vi "PNS Ausgabefelder einfaerben.vi"(6 "Aktionen":T1, 9 "maxLoop":i32=10, 11 "Angehängtes Array":refnum<vi>[](array[refnum])) -> ()   [LabVIEW 2020, in "PNS.lvlib" / "PNS Anlagenuebersicht.lvlib"]
uses:
  PNS Anlagenuebersicht.lvlib
  PNS Ausgabefelder einfaerben Aktionen.ctl
  Aktionen FGV Grenzwerte.ctl
  Allgemein/allgemeine Sub-VIs.lvlib
  PNS.lvlib
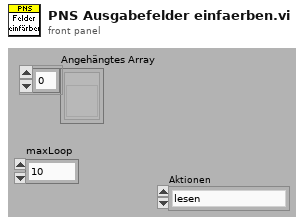
[diagram p1: front panel]
types:
  T1 = typedef "PNS.lvlib/PNS Anlagenuebersicht.lvlib/PNS Ausgabefelder einfaerben Aktionen.ctl" = enum16{"lesen", "prüfen", "initialisieren"}
  T2 = typedef "PNS.lvlib/Aktionen FGV Grenzwerte.ctl" = enum16{"lesen", "Grenzw. schreiben", "Anweisungscode", "IP-Adresse", "laden", "speichern", "Anweisungscode vorgeben"}
  T3 = typedef "Steuerung PNS.lvclass/Anlegengrenzwerte PNS.ctl" = cluster{"Filter:":T4, "Ventilplatte:":T4, "Heizleitung 1:":T4, "Heizleitung 2:":T4, "Heizleitung 3:":T4, "Heizleitung 4:":T4, "Heizleitung 5:":T4, "Heizleitung 6:":T4}
  T4 = typedef "Steuerung PNS.lvclass/Anlagengrenzwerte Parameteranzeige.ctl" = cluster{"Sollwert":T5, "Warn-Min":T5, "Warn-Max":T5, "Abschalt-Min":T5, "Abschalt-Max":T5, "Regler":u16, "AnlagenParameter":string}
  T5 = typedef "Zahlen-Eingabefeld.ctl" = sgl
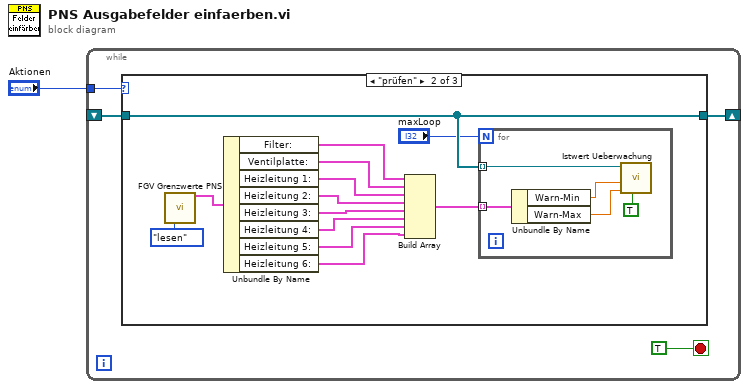
[diagram p0: block diagram]
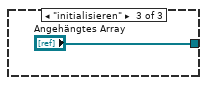
[diagram p3: hidden frame]
diagram:
  n1 = while {
    tunnel: "Aktionen" -> [w5]
    shift-right: [w4] -> _
    shift-left: _ -> [w3]
    stop <- TRUE stop-if-true
    n2 = case shown="\"prüfen\"" w5 {
      tunnel: [w6 w13 "Angehängtes Array"] -> w4
      tunnel: w3 -> [w6 w13 _]
      frame "lesen", Default {
      }
      frame "prüfen" {
        n3 = call "FGV Grenzwerte PNS.vi"("Aktionen FGV Grenzwerte"=Aktionen_FGV_Grenzwerte."lesen") -> ("Grenzwerte PNS 2"=w11:T3)  [unwired: 12 in, 2 out]
        n4 = Unbundle By Name(w11) -> ("Filter:"=w19:T4, "Ventilplatte:"=w18:T4, "Heizleitung 1:"=w17:T4, "Heizleitung 2:"=w16:T4, "Heizleitung 3:"=w15:T4, "Heizleitung 4:"=w10:T4, "Heizleitung 5:"=w9:T4, "Heizleitung 6:"=w8:T4)
        n5 = Build Array(w19, w18, w17, w16, w15, w10, w9, w8) -> (w14:T4[])
        n6 = for {
          N: "maxLoop" -> [_]
          tunnel: w13 -> [w21] mode=indexing
          tunnel: w14 -> [w24] mode=indexing
          n7 = Unbundle By Name(w24) -> ("Warn-Min"=w23:T5, "Warn-Max"=w22:T5)
          n8 = call "Istwert Ueberwachung.vi"("Fehler Aktiviert?"=TRUE, "Max"=w22, "Min"=w23, "Referernz"=w21) -> ()  [unwired: 8 in]
        }
      }
      frame "initialisieren" {
      }
    }
  }
